vi "FlatToRichnixnet_grpc_GetSubPropertyRequest.vi"(5 "OutputClusterType":T1, 11 "InputCluster":T3) -> (3 "OutputCluster":T1)   [LabVIEW 2025, in "grpc-xnet_client.lvlib"]
uses:
  nixnet_grpc_GetSubPropertyRequest_Flat.ctl
  nidevice_grpc_Session_Flat.ctl
  nixnet_grpc_SubProperty.ctl
  nixnet_grpc_GetSubPropertyRequest.ctl
  nixnet_grpc_GetSubPropertyRequest_subproperty_id_enum/nixnet_grpc_GetSubPropertyRequest_subproperty_id_enum.lvclass
  nidevice_grpc_Session.ctl
  grpc-xnet_client.lvlib
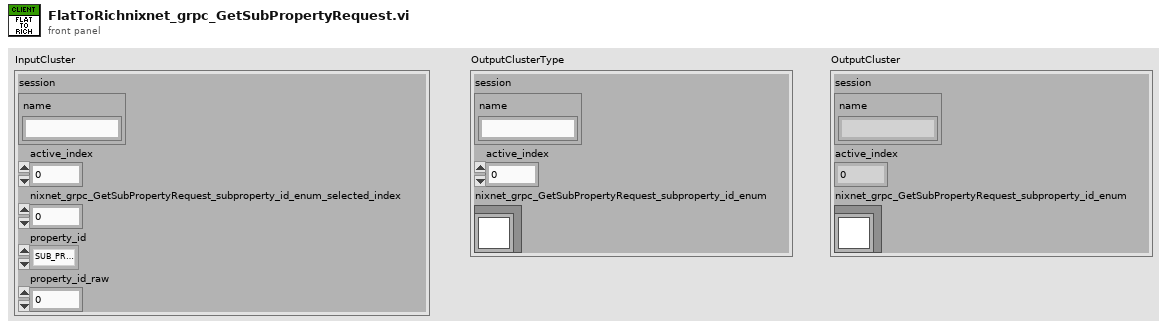
[diagram p1: front panel]
types:
  T1 = typedef "grpc-xnet_client.lvlib/nixnet_grpc_GetSubPropertyRequest.ctl" = cluster{"session":T2, "active_index":u32, "nixnet_grpc_GetSubPropertyRequest_subproperty_id_enum":refnum<class "nixnet_grpc_GetSubPropertyRequest_subproperty_id_enum.lvclass">}
  T2 = typedef "grpc-xnet_client.lvlib/nidevice_grpc_Session.ctl" = cluster{"name":string}
  T3 = typedef "grpc-xnet_client.lvlib/nixnet_grpc_GetSubPropertyRequest_Flat.ctl" = cluster{"session":T4, "active_index":u32, "nixnet_grpc_GetSubPropertyRequest_subproperty_id_enum_selected_index":i32, "property_id":T5, "property_id_raw":u32}
  T4 = typedef "grpc-xnet_client.lvlib/nidevice_grpc_Session_Flat.ctl" = cluster{"name":string}
  T5 = typedef "grpc-xnet_client.lvlib/nixnet_grpc_SubProperty.ctl" = enum32{"SUB_PROPERTY_UNSPECIFIED", "SUB_PROPERTY_SESSION_SUB_CAN_START_TIME_OFF", "SUB_PROPERTY_SESSION_SUB_CAN_TX_TIME", "SUB_PROPERTY_SESSION_SUB_LIN_TX_N_CORRUPTED_CHKSUMS", "SUB_PROPERTY_SESSION_SUB_OUTPUT_QUEUE_UPDATE_FREQ", "SUB_PROPERTY_SESSION_SUB_J1939_ADDR_FILTER", "SUB_PROPERTY_SESSION_SUB_SKIP_N_CYCLIC_FRAMES"}
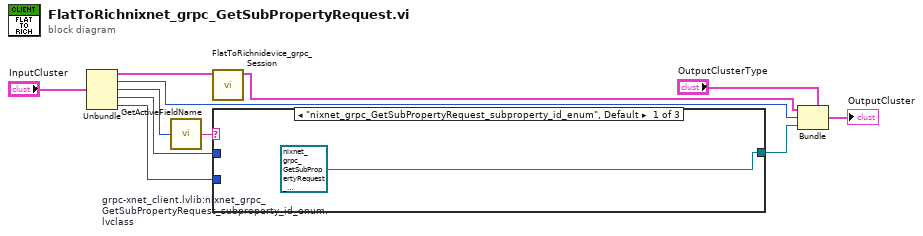
[diagram p0: block diagram]
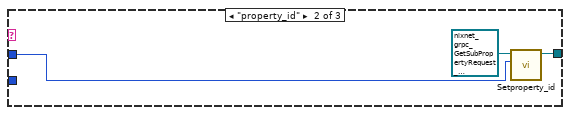
[diagram p2: hidden frame]
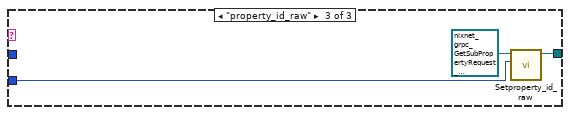
[diagram p3: hidden frame]
diagram:
  n1 = Unbundle "Unbundle"("InputCluster") -> ("session"=w8:T4, "active_index"=w6:u32, "nixnet_grpc_GetSubPropertyRequest_subproperty_id_enum_selected_index"=w5:i32, "property_id"=w2:T5, "property_id_raw"=w1:u32)
  n2 = call "GetActiveFieldName.vi"("protobuf index"=w5) -> ("oneof field name"=w4:string)
  n3 = call "FlatToRichnidevice_grpc_Session.vi"("InputCluster"=w8) -> ("OutputCluster"=w7:T2)  [unwired: 10 in]
  n4 = case "nixnet_grpc_GetSubPropertyRequest_subproperty_id_enum" shown="\"nixnet_grpc_GetSubPropertyRequest_subproperty_id_enum\", Default" w4 {
    tunnel: [w12 w14 w17] -> w3
    tunnel: w2 -> [_ w15 _]
    tunnel: w1 -> [_ _ w18]
    frame "nixnet_grpc_GetSubPropertyRequest_subproperty_id_enum", Default {
      w12 = refnum<class "nixnet_grpc_GetSubPropertyRequest_subproperty_id_enum.lvclass"> refnum  # grpc-xnet_client.lvlib:nixnet_grpc_GetSubPropertyRequest_subproperty_id_enum.lvclass
    }
    frame "property_id" {
      n5 = call "Setproperty_id.vi"("Set_Val"=w15, "OneOfTemplate in"=refnum<class "nixnet_grpc_GetSubPropertyRequest_subproperty_id_enum.lvclass"> refnum) -> ("OneOfTemplate out"=w14:refnum<class "nixnet_grpc_GetSubPropertyRequest_subproperty_id_enum.lvclass">)  [unwired: 8 in, 1 out]
    }
    frame "property_id_raw" {
      n6 = call "Setproperty_id_raw.vi"("Set_Val"=w18, "OneOfTemplate in"=refnum<class "nixnet_grpc_GetSubPropertyRequest_subproperty_id_enum.lvclass"> refnum) -> ("OneOfTemplate out"=w17:refnum<class "nixnet_grpc_GetSubPropertyRequest_subproperty_id_enum.lvclass">)  [unwired: 8 in, 1 out]
    }
  }
  n7 = Bundle "Bundle"(cluster="OutputClusterType", "session"=w7, "active_index"=w6, "nixnet_grpc_GetSubPropertyRequest_subproperty_id_enum"=w3) -> (→"OutputCluster":T1)
